vi "Save parameters to file.vi"(8 "error in":errorcluster, 11 "Config":T1={"DAQ"={"Data"={"Live"={"t0"=timestamp(0 s since 1904-01-01), "dt"=1.0, "Y"=[]}, "Accumulated"={"t0"=timestamp(0 s since 1904-01-01), "dt"=1.0, "Y"=[]}, "Averaged"={"t0"=timestamp(0 s since 1904-01-01), "dt"=1.0, "Y"=[]}, "data array"=[], "live time array"=[], "Live (decimated)"={"t0"=timestamp(0 s since 1904-01-01), "dt"=1.0, "Y"=[]}}, "Config"={"Input Config"=10106, "Card"=enum."USB-6211", "100% Reflectance Standard (V)"=1.0, "Input Channel"="Dev2/ai0", "Average number of points"=50.0, "Trigger Level (V)"=0.4, "Rate (Hz)"=250000, "End Time (s)"=1.0}, "Indicators"={"Final number of points"=0.0, "Number of samples"=0.0, "dt"=0.0, "Shots"=1, "Shot counter"=0, "Test counter"=0, "Background level (V)"=0.0, "DAQ task"="", "timestamp of data"=timestamp(0 s since 1904-01-01), "Test Type"=enum."A-Test"}}, "Shutter"={"Open command string"="", "VISA"={"Timeout (ms)"=0, "Resource Name"="", "Baud Rate"=0, "Data Bits"=0, "Parity"=0, "Stop Bits"=0, "Flow Control"=0}}, "Monochromator"={"Type"=enum."Oriel", "Wavelength (nm)"=0.0, "Grating, gr/mm"=enum."2400", "Grating mode"=enum."Unknown", "Spectrum mode"={"Spectrum mode?"=FALSE, "Start wavelength (nm)"=0.0, "End wavelength (nm)"=0.0, "Wavelength step (nm)"=0.0, "Wavelength array"=[], "array index"=0}, "PTI"={"Delay before read (ms)"=0, "Mono 1"={"Timeout (ms)"=0, "Resource Name"="", "Baud Rate"=0, "Data Bits"=0, "Parity"=0, "Stop Bits"=0, "Flow Control"=0}, "Mono 2"={"Timeout (ms)"=0, "Resource Name"="", "Baud Rate"=0, "Data Bits"=0, "Parity"=0, "Stop Bits"=0, "Flow Control"=0}, "Two PTI Monochromators?"=FALSE}, "Oriel (custom)"={"reference"=refnum}, "Force wavelength confirmation (PTI)?"=FALSE}, "Test"={"Config"={"Amplification Factor"=0.0, "100% Reflectance Standard"=0.0, "Calculation Method"=enum."Reflectance", "Option to discard new data?"=FALSE, "Mode"=enum."Spectrum", "Number of Averages"=0, "B Test?"=FALSE}, "Indicators"={"DAQ Background Level (V)"=0.0, "A-Test Counter"=0, "B-Test Counter"=0, "Type"=enum."A-Test", "Scope Background Level (Amps)"=2.0, "TAS only?"=FALSE}}, "Scope"={"Config"={"VISA Resource"="USB0::0x0699::0x039D::C010764::INSTR", "Model"=enum."DPO 2012B", "Timebase"=0.0004, "Timeout (ms)"=60000, "TAS"={"Vertical Range (V)"=2.0, "Vertical Offset (0.0 divs)"=0.0, "Bandwidth"=0, "Probe Attenuation (10.0)"=1.0, "Vertical Coupling"=1, "Impedance"=0, "Multiplication factor"=1.0, "Channel"=enum."Channel 1"}, "TPC"={"Vertical Range (V)"=2.0, "Vertical Offset (0.0 divs)"=0.0, "Bandwidth"=0, "Probe Attenuation (10.0)"=1.0, "Vertical Coupling"=1, "Impedance"=0, "Multiplication factor"=1.0, "Channel"=enum."None"}, "Trigger"={"Mode"=enum."Laser (TAS)", "Source "=enum."Aux", "PIA"={"Test LEDs"=FALSE, "LED line"="", "LED off (s)"=0.0, "LED on (s)"=0.0}, "Threshold (V)"=0.8}}, "Indicators"={"Setup"={"Final number of points"=0.0, "Pretrigger points"=0.0, "Number of readouts"=0, "Model"={"Acquisition Type"=4, "Record length (points)"=1000, "Averages on scope"=4, "Average number of points"=10.0}}, "Timestamp of Data"=timestamp(0 s since 1904-01-01)}, "Data"={"TPC"={"Live data"={"t0"=timestamp(0 s since 1904-01-01), "dt"=1.0, "Y"=[]}, "Averaged data"={"t0"=timestamp(0 s since 1904-01-01), "dt"=1.0, "Y"=[]}, "Accumulated data"={"t0"=timestamp(0 s since 1904-01-01), "dt"=1.0, "Y"=[]}, "Final data"={"t0"=timestamp(0 s since 1904-01-01), "dt"=1.0, "Y"=[]}}, "TAS"={"Live data"={"t0"=timestamp(0 s since 1904-01-01), "dt"=1.0, "Y"=[]}, "Averaged data"={"t0"=timestamp(0 s since 1904-01-01), "dt"=1.0, "Y"=[]}, "Accumulated data"={"t0"=timestamp(0 s since 1904-01-01), "dt"=1.0, "Y"=[]}, "Final data"={"t0"=timestamp(0 s since 1904-01-01), "dt"=1.0, "Y"=[]}}, "Time arrays"={"Time array (decimated)"=[], "waveform"={"t0"=timestamp(0 s since 1904-01-01), "dt"=1.0, "Y"=[]}}}, "Test"={"Config"={"Amplification Factor"=0.0, "100% Reflectance Standard"=0.0, "Calculation Method"=enum."Reflectance", "Option to discard new data?"=FALSE, "Mode"=enum."Spectrum", "Number of Averages"=100, "B Test?"=FALSE}, "Indicators"={"DAQ Background Level (V)"=2.0, "A-Test Counter"=2, "B-Test Counter"=2, "Type"=enum."A-Test", "Scope Background Level (Amps)"=2.0, "TAS only?"=FALSE}}}, "Colour wheel"={"Reference"=0, "Colour Wheel Wavelengths"=[], "Waveform Index"=0, "COM Port"="", "Enabled?"=FALSE}, "File IO"={"Output Folder"=path "C:/Users/Abigail/Documents/Imperial Optical software/Optical Software Code Simplified/Output", "Error file"=path "C:/Users/Abigail/Documents/Imperial Optical software/Optical Software Code Simplified/Error Log.txt", "Config file"=path "C:/Users/Abigail/Documents/Imperial Optical software/Optical Software Code Simplified/Config.ini", "File prefix"="", "Waveform read"={"t0"=timestamp(0 s since 1904-01-01), "dt"=1.0, "Y"=[]}}} {"Scope"."Test"."Config"."Number of Averages" min=0; "Scope"."Indicators"."Setup"."Model"."Record length (points)" items=["1000"=1, "10,000"=10, "100,000"=100, "1,000,000"=1000, "5,000,000"=5000, "10,000,000"=10000]; "Scope"."Indicators"."Setup"."Model"."Acquisition Type" items=["Sample", "Peak Detect", "Hi Res", "Envelope", "Average"]; "Scope"."Config"."Trigger"."Threshold (V)" format="%#_3f"; "Scope"."Config"."TPC"."Impedance" items=["1M", "75", "50"]; "Scope"."Config"."TPC"."Vertical Coupling" items=["AC", "DC", "Ground"]; "Scope"."Config"."TPC"."Bandwidth" items=["FULL", "250 MHz", "150 MHz", "20 MHz"]; "Scope"."Config"."TAS"."Impedance" items=["1M", "75", "50"]; "Scope"."Config"."TAS"."Vertical Coupling" items=["AC", "DC", "Ground"]; "Scope"."Config"."TAS"."Bandwidth" items=["FULL", "250 MHz", "150 MHz", "20 MHz"]; "Scope"."Config"."Timebase" format="%^#_3e"; "Test"."Config"."Number of Averages" min=0; "Monochromator"."PTI"."Mono 2"."Flow Control" items=["1.0"=10, "1.5"=15, "2.0"=20]; "Monochromator"."PTI"."Mono 2"."Stop Bits" items=["None", "Odd", "Even", "Mark", "Space"]; "Monochromator"."PTI"."Mono 2"."Parity" items=["None", "Odd", "Even", "Mark", "Space"]; "Monochromator"."PTI"."Mono 1"."Flow Control" items=["1.0"=10, "1.5"=15, "2.0"=20]; "Monochromator"."PTI"."Mono 1"."Stop Bits" items=["None", "Odd", "Even", "Mark", "Space"]; "Monochromator"."PTI"."Mono 1"."Parity" items=["None", "Odd", "Even", "Mark", "Space"]; "Shutter"."VISA"."Flow Control" items=["None"=0, "XON/XOFF"=1, "RTS/CTS"=2, "DTR/DSR"=4]; "Shutter"."VISA"."Stop Bits" items=["1.0"=10, "1.5"=15, "2.0"=20]; "Shutter"."VISA"."Parity" items=["None", "Odd", "Even", "Mark", "Space"]; "DAQ"."Config"."Input Config" items=["default"=-1, "RSE"=10083, "NRSE"=10078, "Differential"=10106, "Pseudodifferential"=12529]}) -> (0 "error out":errorcluster)   [LabVIEW 2017, in "File IO.lvlib"]
uses:
  File IO.lvlib
  System Control/CTLs/Params.ctl
  DAQ/Controls/Params.ctl
  DAQ/Controls/DAQ Config.ctl
  DAQ/Controls/DAQ Indicators.ctl
  System Control/CTLs/Test Type.ctl
  Shutter Module/Controls/Params.ctl
  Monochromator/Controls/VISA parameters.ctl
  Monochromator/Controls/Params.ctl
  Monochromator/Controls/Type.ctl
  Monochromator/Controls/GratingValues.ctl
  Monochromator/Controls/Grating.ctl
  Monochromator/PTI/Controls/Params.ctl
  Monochromator/Custom Oriel drivers/Controls/Params.ctl
  C:/Project Work/icl-optical-software-rewrite/Optical Software Code Simplified/Modules/Monochromator/Cornerstone.dll
  Monochromator/Cornerstone.dll
  System Control/CTLs/Test params.ctl
  System Control/CTLs/Test Controls.ctl
  System Control/CTLs/Test indicators.ctl
  Scope/Controls/Params.ctl
  Scope/Controls/Models.ctl
  Scope/Controls/TPC.ctl
  Scope/Controls/Channels.ctl
  Trigger/Controls/Params.ctl
  Trigger/Controls/Mode.ctl
  Trigger/Controls/Trigger channels.ctl
  Scope/Controls/Acquisition type.ctl
  Scope/Controls/Record length.ctl
  Scope/Controls/Data.ctl
  Scope/Controls/Channel data.ctl
  Colour Wheel/Controls/Params.ctl
  Controls/Params.ctl
  DAQ/DAQ.lvlib
  Serial comms/Serial comms.lvlib
  Shutter Module/Shutter.lvlib
  Monochromator/Monochromator.lvlib
  Monochromator/PTI/PTI.lvlib
  Monochromator/Custom Oriel drivers/Oriel (custom drivers).lvlib
  System Control/Main controller.lvlib
  Scope/Scope.lvlib
  Trigger/Trigger.lvlib
  Colour Wheel/Colour Wheel.lvlib
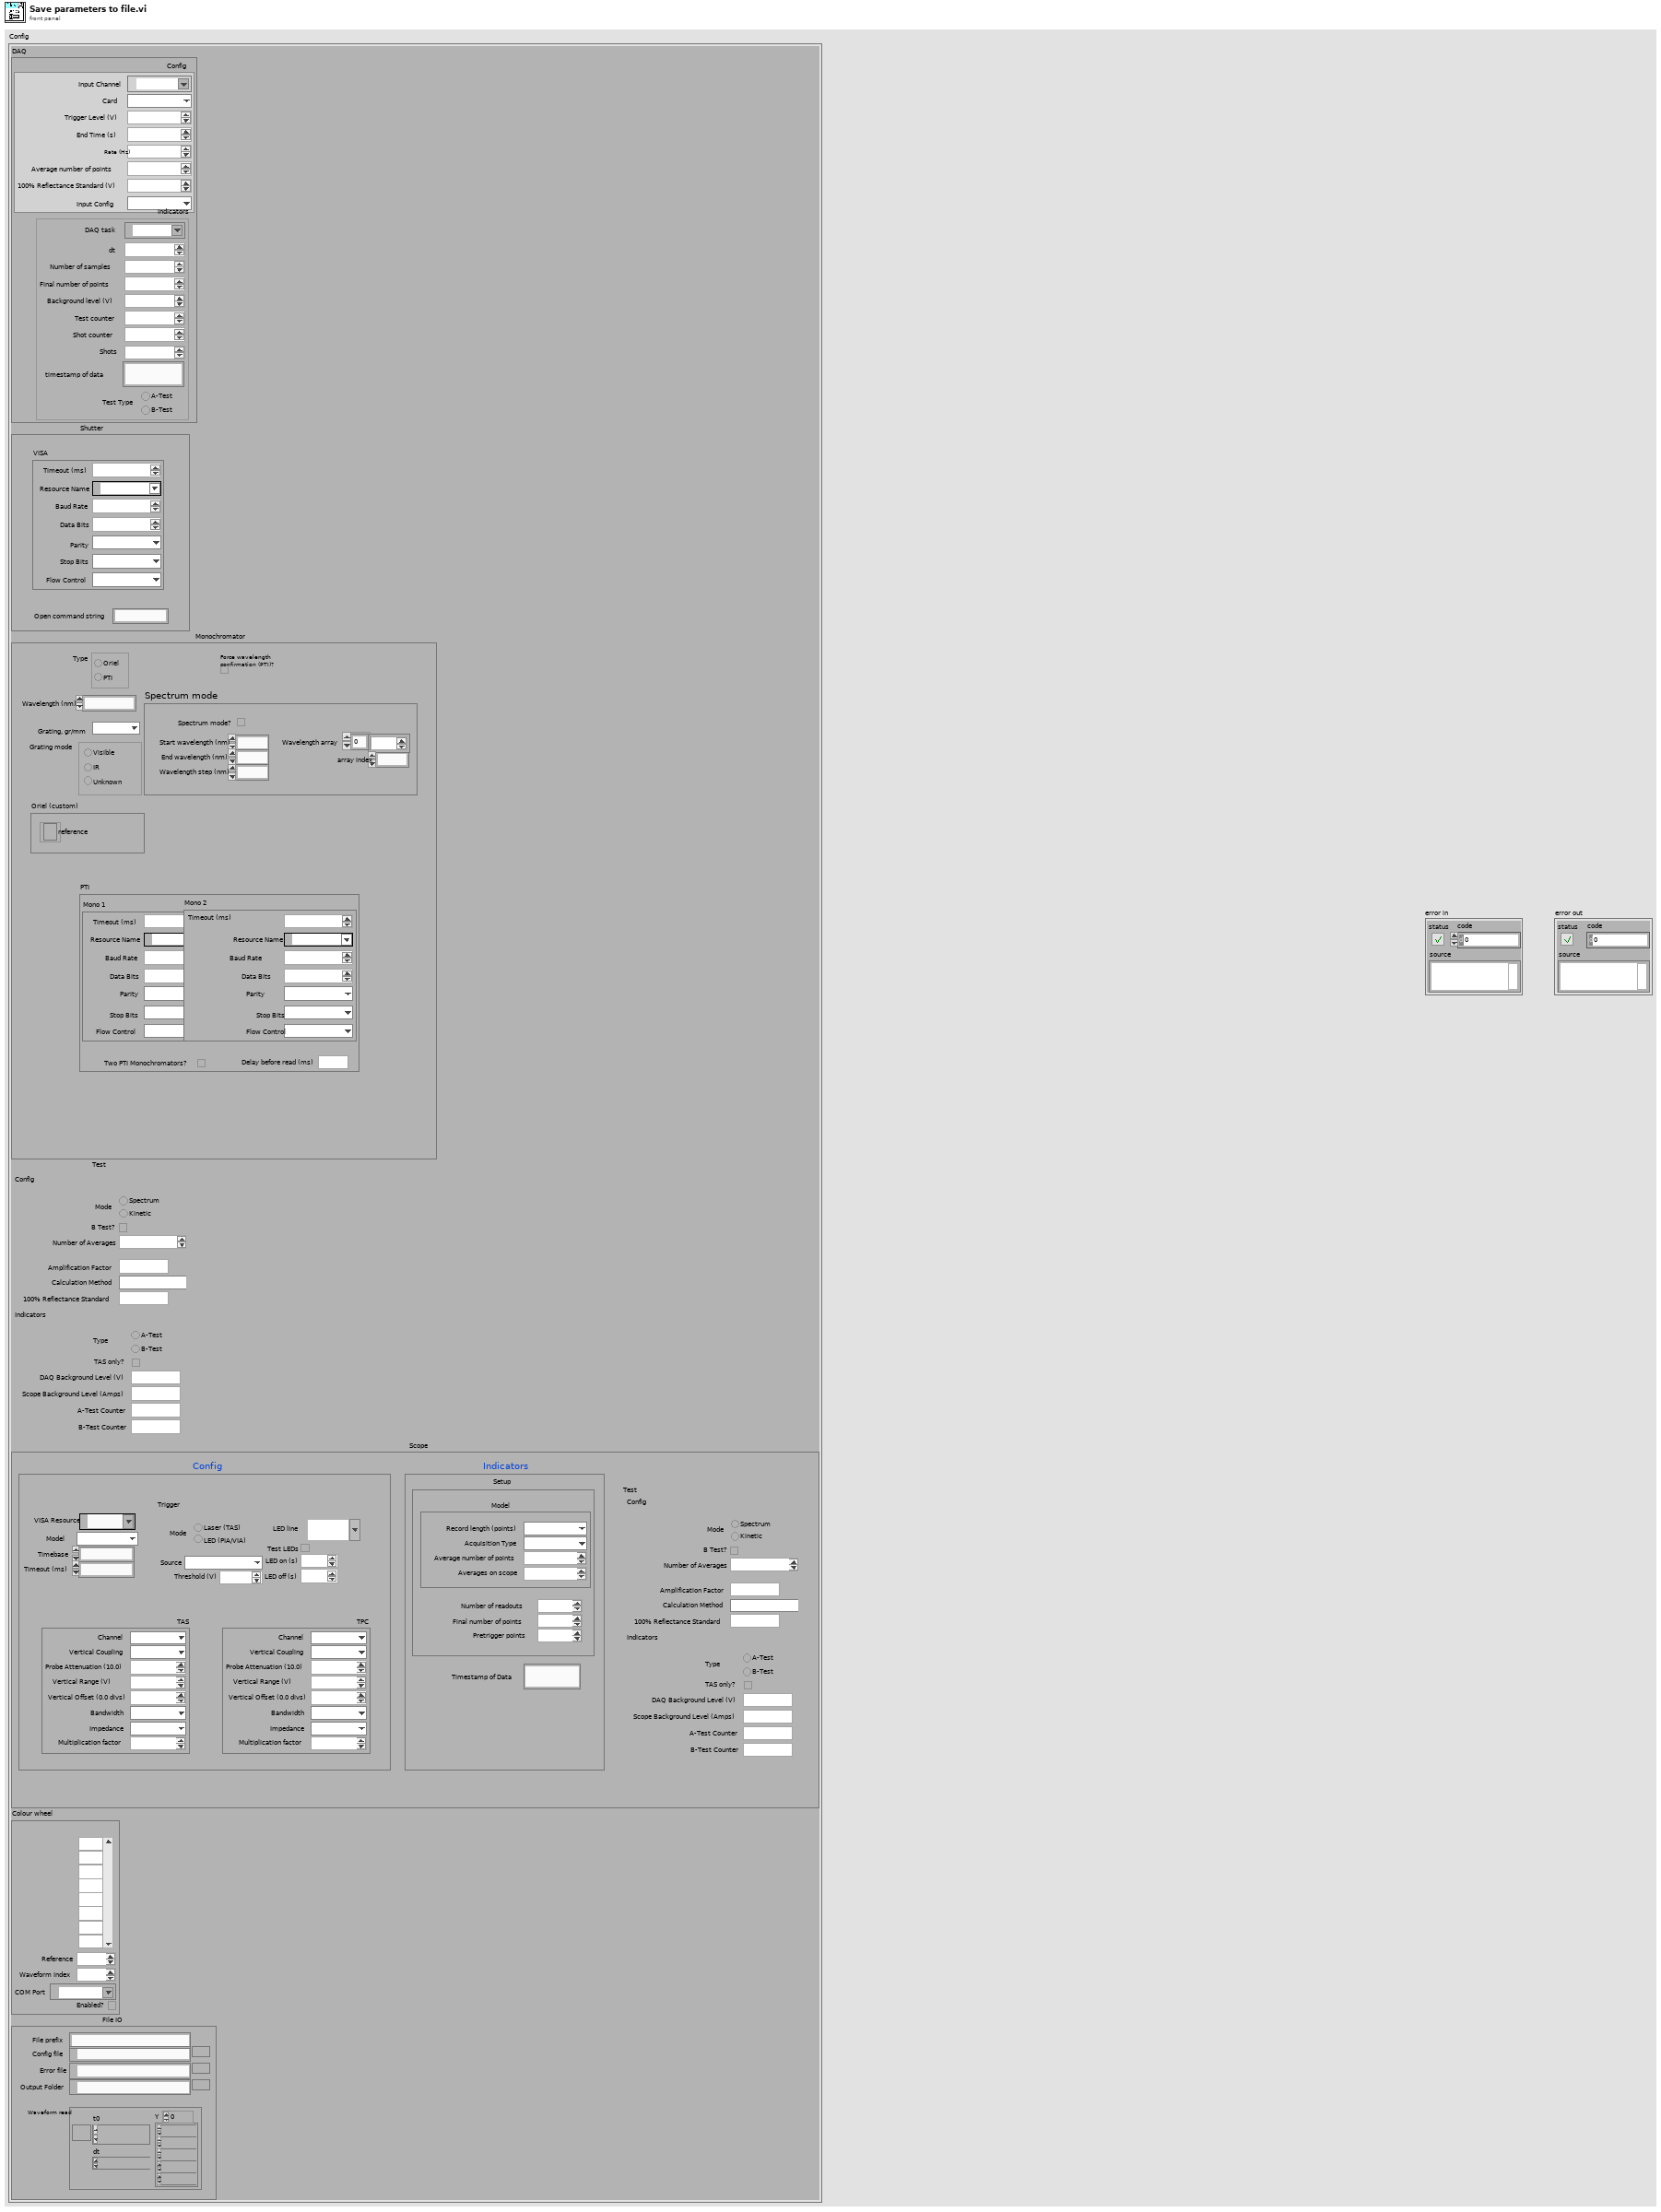
[diagram p1: front panel]
types:
  T1 = typedef "Main controller.lvlib/Params.ctl" = cluster{"DAQ":T2, "Shutter":T6, "Monochromator":T8, "Test":T14, "Scope":T17, "Colour wheel":T28, "File IO":T29}
  T2 = typedef "DAQ.lvlib/Params.ctl" = cluster{"Data":cluster{"Live":waveform(dbl), "Accumulated":waveform(dbl), "Averaged":waveform(dbl), "data array":dbl[], "live time array":dbl[], "Live (decimated)":waveform(dbl)}, "Config":T3, "Indicators":T4}
  T3 = typedef "DAQ.lvlib/DAQ Config.ctl" = cluster{"Input Config":i32, "Card":enum16{"USB-6211", "USB-6251", "USB-6361"}, "100% Reflectance Standard (V)":dbl, "Input Channel":tag, "Average number of points":dbl, "Trigger Level (V)":dbl, "Rate (Hz)":i32, "End Time (s)":dbl}
  T4 = typedef "DAQ.lvlib/DAQ Indicators.ctl" = cluster{"Final number of points":dbl, "Number of samples":dbl, "dt":dbl, "Shots":i32, "Shot counter":i32, "Test counter":i32, "Background level (V)":dbl, "DAQ task":refnum<k21>, "timestamp of data":timestamp, "Test Type":T5}
  T5 = typedef "Main controller.lvlib/Test Type.ctl" = enum32{"A-Test", "B-Test"}
  T6 = typedef "Shutter.lvlib/Params.ctl" = cluster{"Open command string":string, "VISA":T7}
  T7 = typedef "Serial comms.lvlib/VISA parameters.ctl" = cluster{"Timeout (ms)":u32, "Resource Name":refnum<visa-resource-name>, "Baud Rate":u32, "Data Bits":u16, "Parity":u16, "Stop Bits":u16, "Flow Control":u16}
  T8 = typedef "Monochromator.lvlib/Params.ctl" = cluster{"Type":T9, "Wavelength (nm)":dbl, "Grating, gr/mm":T10, "Grating mode":T11, "Spectrum mode":cluster{"Spectrum mode?":bool, "Start wavelength (nm)":dbl, "End wavelength (nm)":dbl, "Wavelength step (nm)":dbl, "Wavelength array":dbl[], "array index":u32}, "PTI":T12, "Oriel (custom)":T13, "Force wavelength confirmation (PTI)?":bool}
  T9 = typedef "Monochromator.lvlib/Type.ctl" = enum32{"Oriel", "PTI"}
  T10 = typedef "Monochromator.lvlib/GratingValues.ctl" = enum16{"2400", "1800", "1200", "600", "300", "150"}
  T11 = typedef "Monochromator.lvlib/Grating.ctl" = enum32{"Unknown", "Visible", "IR"}
  T12 = typedef "Monochromator.lvlib/PTI.lvlib/Params.ctl" = cluster{"Delay before read (ms)":u32, "Mono 1":T7, "Mono 2":T7, "Two PTI Monochromators?":bool}
  T13 = typedef "Monochromator.lvlib/Oriel (custom drivers).lvlib/Params.ctl" = cluster{"reference":refnum<k24>}
  T14 = typedef "Main controller.lvlib/Test params.ctl" = cluster{"Config":T15, "Indicators":T16}
  T15 = typedef "Main controller.lvlib/Test Controls.ctl" = cluster{"Amplification Factor":dbl, "100% Reflectance Standard":dbl, "Calculation Method":enum16{"Reflectance", "Transmission", "Kubelka-Munk"}, "Option to discard new data?":bool, "Mode":enum32{"Spectrum", "Kinetic"}, "Number of Averages":i32, "B Test?":bool}
  T16 = typedef "Main controller.lvlib/Test indicators.ctl" = cluster{"DAQ Background Level (V)":dbl, "A-Test Counter":i32, "B-Test Counter":i32, "Type":T5, "Scope Background Level (Amps)":dbl, "TAS only?":bool}
  T17 = typedef "Scope.lvlib/Params.ctl" = cluster{"Config":cluster{"VISA Resource":refnum<visa-resource-name>, "Model":T18, "Timebase":dbl, "Timeout (ms)":u32, "TAS":T19, "TPC":T19, "Trigger":T21}, "Indicators":cluster{"Setup":cluster{"Final number of points":dbl, "Pretrigger points":dbl, "Number of readouts":i32, "Model":cluster{"Acquisition Type":T24, "Record length (points)":T25, "Averages on scope":i32, "Average number of points":dbl}}, "Timestamp of Data":timestamp}, "Data":T26, "Test":T14}
  T18 = typedef "Scope.lvlib/Models.ctl" = enum16{"DPO 3012", "DPO 2012B", "TDS 3012C"}
  T19 = typedef "Scope.lvlib/TPC.ctl" = cluster{"Vertical Range (V)":dbl, "Vertical Offset (0.0 divs)":dbl, "Bandwidth":i32, "Probe Attenuation (10.0)":dbl, "Vertical Coupling":u16, "Impedance":u16, "Multiplication factor":dbl, "Channel":T20}
  T20 = typedef "Scope.lvlib/Channels.ctl" = enum16{"Channel 1", "Channel 2", "Channel 3", "Channel 4", "Math", "Reference A", "Reference B", "Reference C", "Reference D", "B1", "B2", "None"}
  T21 = typedef "Scope.lvlib/Trigger.lvlib/Params.ctl" = cluster{"Mode":T22, "Source ":T23, "PIA":cluster{"Test LEDs":bool, "LED line":tag, "LED off (s)":dbl, "LED on (s)":dbl}, "Threshold (V)":dbl}
  T22 = typedef "Scope.lvlib/Trigger.lvlib/Mode.ctl" = enum32{"Laser (TAS)", "LED (PIA/VIA)"}
  T23 = typedef "Scope.lvlib/Trigger.lvlib/Trigger channels.ctl" = enum16{"Channel 1", "Channel 2", "Channel 3", "Channel 4", "AC Line", "Aux", "Digital Channel 0", "Digital Channel 1", "Digital Channel 2", "Digital Channel 3", "Digital Channel 4", "Digital Channel 5", "Digital Channel 6", "Digital Channel 7", "Digital Channel 8", "Digital Channel 9", "Digital Channel 10", "Digital Channel 11", "Digital Channel 12", "Digital Channel 13", "Digital Channel 14", "Digital Channel 15", "RF"}
  T24 = typedef "Scope.lvlib/Acquisition type.ctl" = u16
  T25 = typedef "Scope.lvlib/Record length.ctl" = u32
  T26 = typedef "Scope.lvlib/Data.ctl" = cluster{"TPC":T27, "TAS":T27, "Time arrays":cluster{"Time array (decimated)":dbl[], "waveform":waveform(dbl)}}
  T27 = typedef "Scope.lvlib/Channel data.ctl" = cluster{"Live data":waveform(dbl), "Averaged data":waveform(dbl), "Accumulated data":waveform(dbl), "Final data":waveform(dbl)}
  T28 = typedef "Colour Wheel.lvlib/Params.ctl" = cluster{"Reference":i32, "Colour Wheel Wavelengths":dbl[], "Waveform Index":i32, "COM Port":refnum<visa-resource-name>, "Enabled?":bool}
  T29 = typedef "File IO.lvlib/Params.ctl" = cluster{"Output Folder":path, "Error file":path, "Config file":path, "File prefix":string, "Waveform read":waveform(dbl)}
  T30 = enum16{"Reflectance", "Transmission", "Kubelka-Munk"}
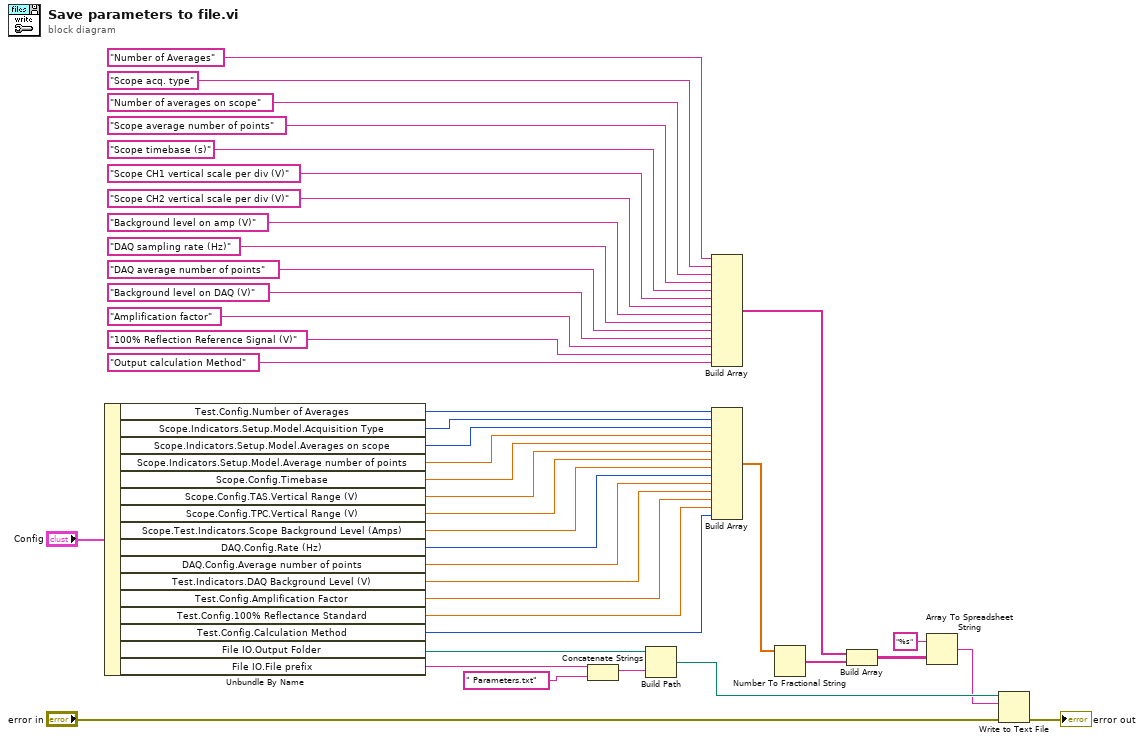
[diagram p0: block diagram]
diagram:
  n1 = Unbundle By Name("Config") -> ("Test.Config.Number of Averages"=w28:i32, "Scope.Indicators.Setup.Model.Acquisition Type"=w29:T24, "Scope.Indicators.Setup.Model.Averages on scope"=w30:i32, "Scope.Indicators.Setup.Model.Average number of points"=w31:dbl, "Scope.Config.Timebase"=w32:dbl, "Scope.Config.TAS.Vertical Range (V)"=w33:dbl, "Scope.Config.TPC.Vertical Range (V)"=w34:dbl, "Scope.Test.Indicators.Scope Background Level (Amps)"=w35:dbl, "DAQ.Config.Rate (Hz)"=w36:i32, "DAQ.Config.Average number of points"=w37:dbl, "Test.Indicators.DAQ Background Level (V)"=w38:dbl, "Test.Config.Amplification Factor"=w39:dbl, "Test.Config.100% Reflectance Standard"=w40:dbl, "Test.Config.Calculation Method"=w41:T30, "File IO.Output Folder"=w1:path, "File IO.File prefix"=w2:string)
  n2 = Concatenate Strings(w2, " Parameters.txt") -> (w26:string)
  n3 = Build Path(base path=w1, name or relative path=w26) -> (appended path=w12:path)
  n4 = Build Array("Number of Averages", "Scope acq. type", "Number of averages on scope", "Scope average number of points", "Scope timebase (s)", "Scope CH1 vertical scale per div (V)", "Scope CH2 vertical scale per div (V)", "Background level on amp (V)", "DAQ sampling rate (Hz)", "DAQ average number of points", "Background level on DAQ (V)", "Amplification factor", "100% Reflection Reference Signal (V)" ("element"), "Output calculation Method" ("element")) -> (w14:string[])
  n5 = Build Array(w28, w29, w30, w31, w32, w33, w34, w35, w36, w37, w38, w39, w40, w41) -> (w13:dbl[])
  n6 = Number To Fractional String(number=w13) -> (F-format string=w27:string[])  [unwired: 3 in]
  n7 = Build Array(w14, w27) -> (w11:string[][])
  n8 = Array To Spreadsheet String(array=w11, 3:"%s" ("format string")) -> (spreadsheet string=w9:string)  [unwired: 1 in]
  n9 = Write to Text File(file (use dialog)=w12, text=w9, error in="error in") -> (error out=→"error out":errorcluster)  [unwired: 1 in, 2 out]
